vi "1ALABVIEW.vi"() -> ()   [LabVIEW 2013]
panel:
  out "SQUARE ROOT":dbl
  out "SQUARE":dbl
  out "DIVISION":dbl
  out "MULTIPLACTION":dbl
  out "SUBTRACTION":dbl
  out "ADDITION":dbl
  in  "B":dbl
  in  "A":dbl
  # "1(A).BASIC  ARITHMETIC OPERATIONS"
  # "O.SRINIVAS\n23A91A04H6"
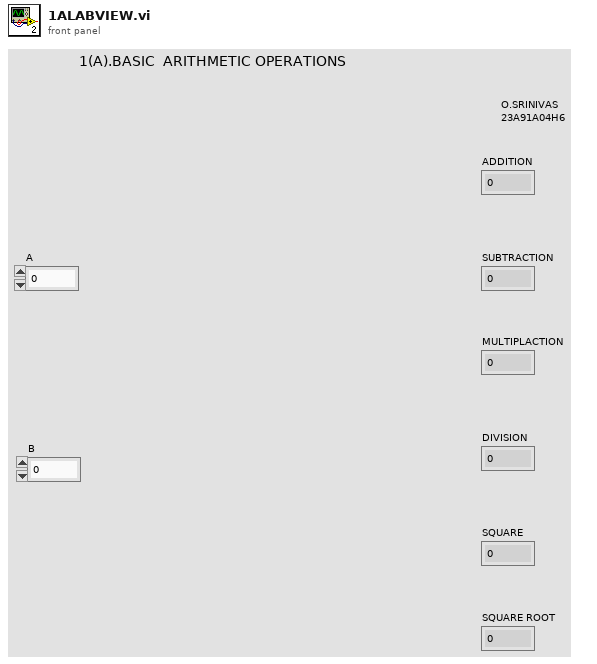
[diagram p1: front panel]
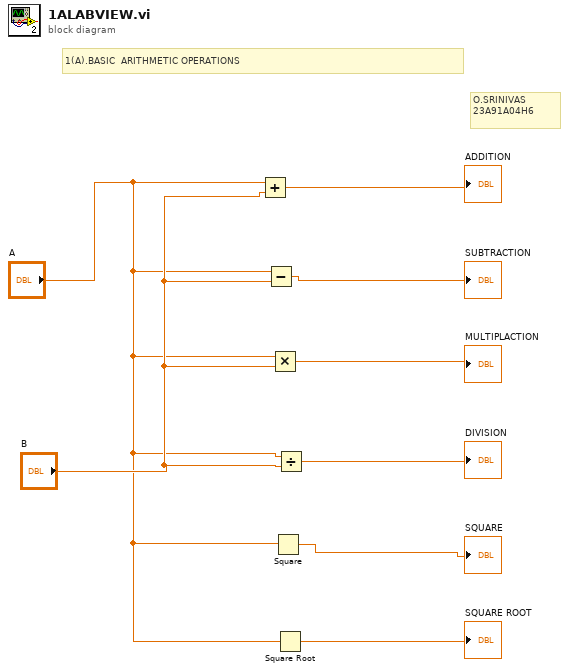
[diagram p0: block diagram]
diagram:
  # "O.SRINIVAS\n23A91A04H6"
  # "1(A).BASIC  ARITHMETIC OPERATIONS"
  n1 = Add(x="A", y="B") -> (x+y=→"ADDITION":dbl)
  n2 = Subtract(x="A", y="B") -> (x-y=→"SUBTRACTION":dbl)
  n3 = Multiply(x="A", y="B") -> (x*y=→"MULTIPLACTION":dbl)
  n4 = Square(x="A") -> (x^2=→"SQUARE":dbl)
  n5 = Square Root(x="A") -> (sqrt(x)=→"SQUARE ROOT":dbl)
  n6 = Divide(x="A", y="B") -> (x/y=→"DIVISION":dbl)
